vi "CAN_LIN_AsynCall.vi"() -> ()   [LabVIEW 2014]
uses:
  <vilib>/Utility/miscctls.llb/LVPointTypeDef.ctl
  CAN_LIN_FlexRay/TypDef/CAN_LIN_FlexRay_Data.ctl
  TypDef/CAN_LIN_Data.ctl
panel:
  in  "DLL_PATH":path=path "D:/Program Files (x86)/TOSUN/TSMaster/bin/TSMaster.dll"
  out "out put":T1={"Communication message"={"Sender"="", "receiver"="", "message"="", "data"=variant}, "Receive data"="", "error in"={"status"=FALSE, "code"=0, "source"=""}, "Data"={"DLL_PATH"=path "", "Call Array"=["CAN_Demo0", "LIN_Demo0"], "Project_PATH"=path ""}, "AsynCall?"=FALSE}
  in  "选项卡控件":enum32{"CAN", "LIN"}(tab)
  in  "Config":bool
  in  "Connect":bool
  in  "Disconnect":bool
  out "Connect ?":bool
  in  "Creat error":bool
  in  "log":i32(listbox)
  in  "Quit":bool
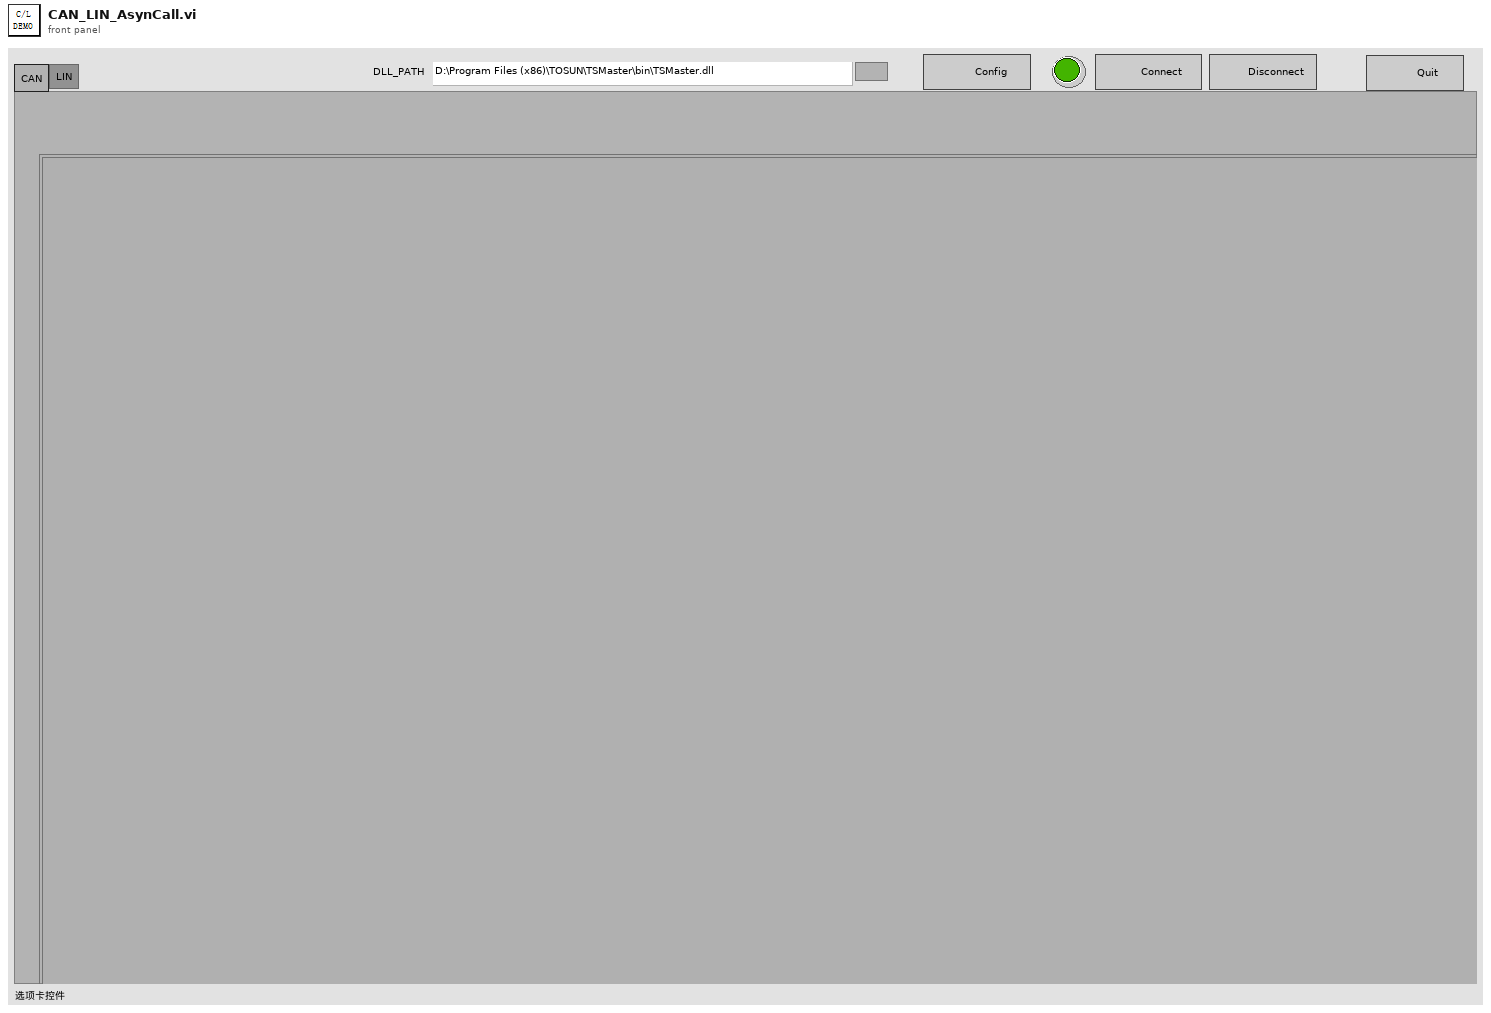
[diagram p1: front panel]
types:
  T1 = typedef "CAN_LIN_Data.ctl" = cluster{"Communication message":cluster{"Sender":string, "receiver":string, "message":string, "data":variant}, "Receive data":string, "error in":errorcluster, "Data":cluster{"DLL_PATH":path, "Call Array":string[], "Project_PATH":path}, "AsynCall?":bool}
  T2 = cluster{"Sender":string, "receiver":string, "message":string, "data":variant}
  T3 = typedef "CAN_LIN_FlexRay_Data.ctl" = cluster{"Communication message":cluster{"Sender":string, "receiver":string, "message":string, "data":variant}, "Receive data":string, "error in":errorcluster, "Data":cluster{"DLL_PATH":path, "Call Array":string[], "Project_PATH":path}, "AsynCall?":bool}
  T4 = typedef "LVPointTypeDef.ctl" = cluster{"Horizontal":i16, "Vertical":i16}
  T5 = enum32{"invalid app kind", "Development System", "Run Time System", "Student Edition", "Embedded LabVIEW", "Evaluation", "Custom"}
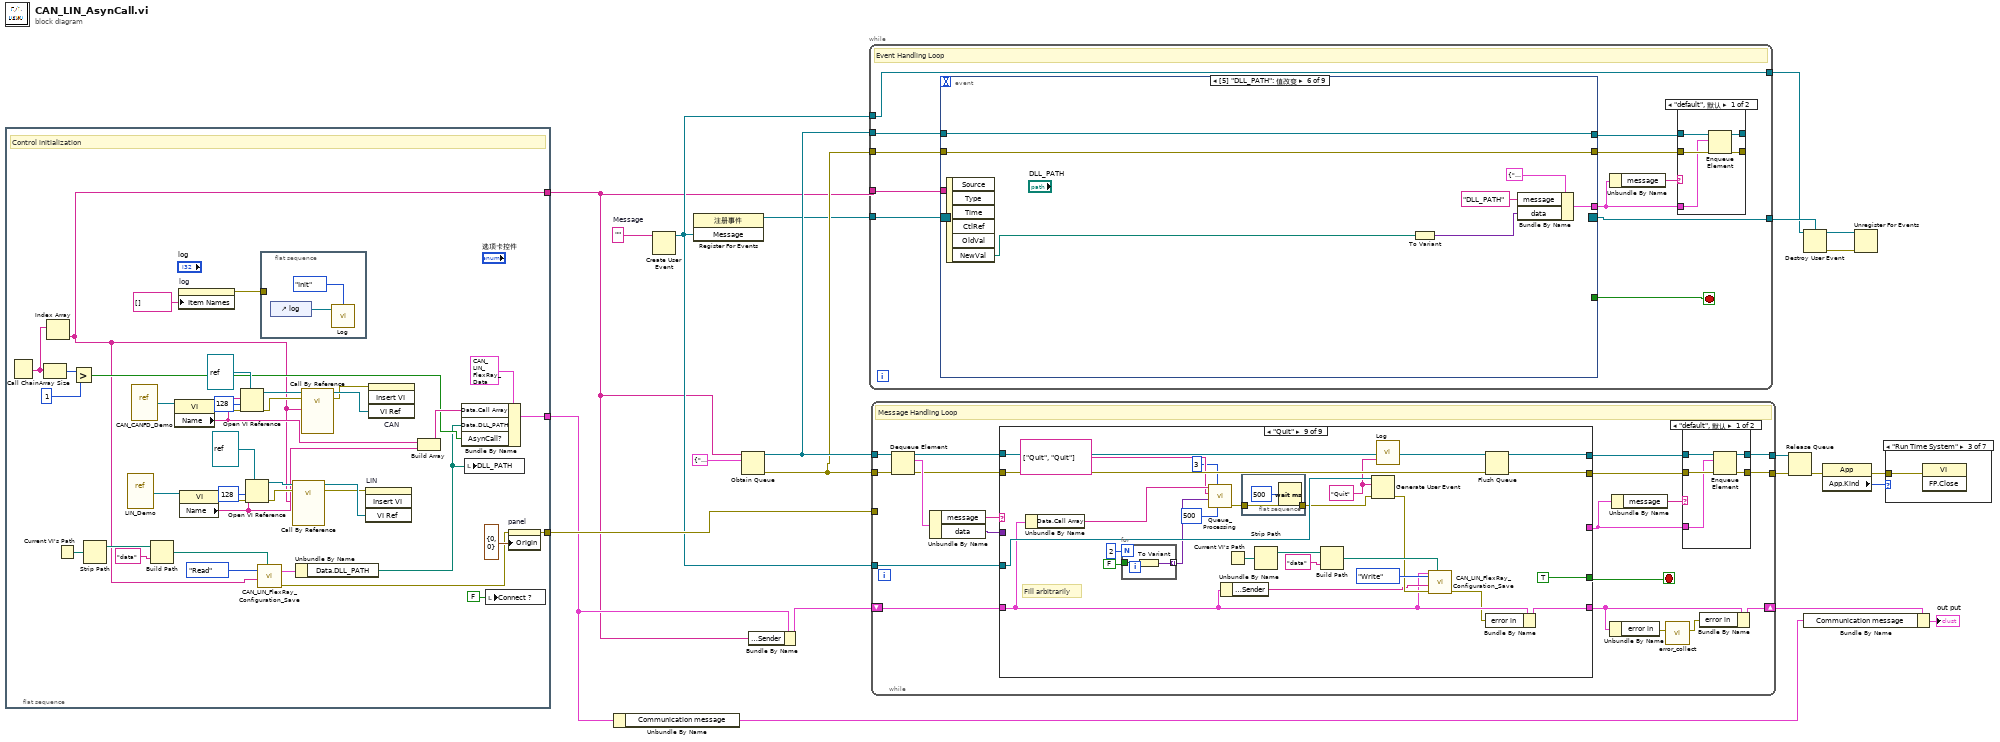
[diagram p0: block diagram]
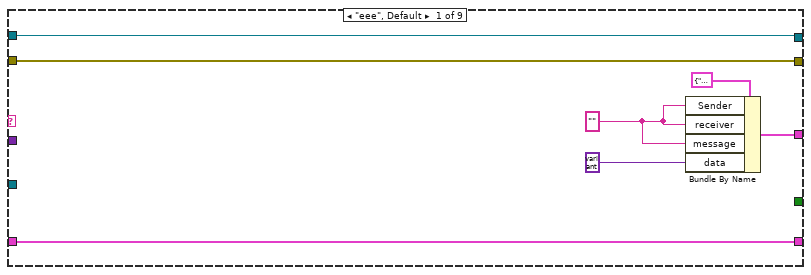
[diagram p9: hidden frame]
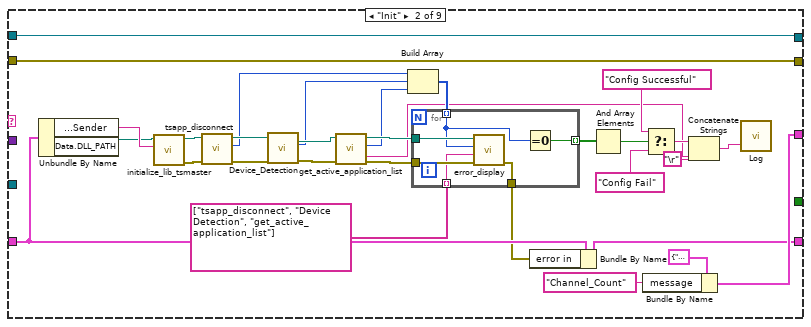
[diagram p10: hidden frame]
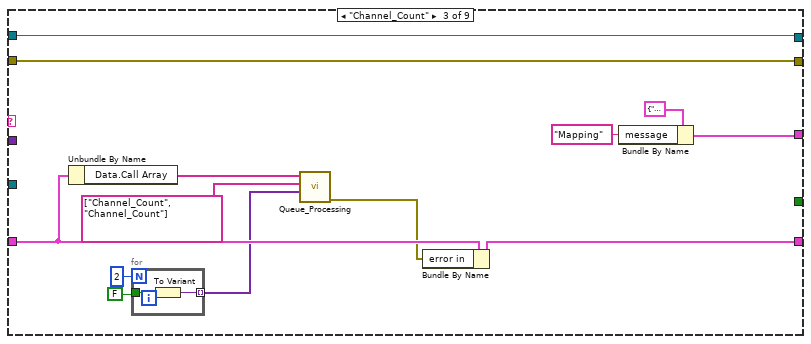
[diagram p11: hidden frame]
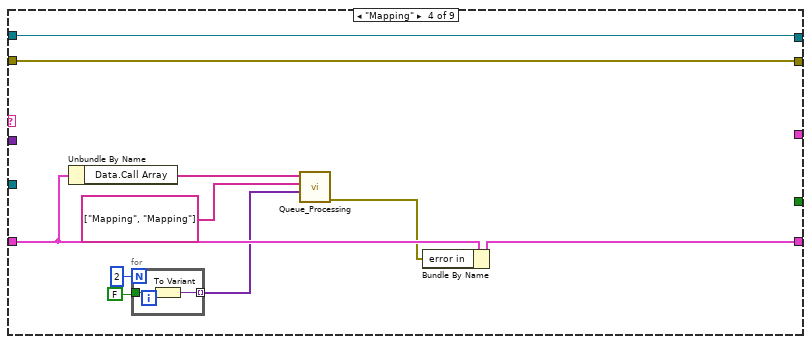
[diagram p12: hidden frame]
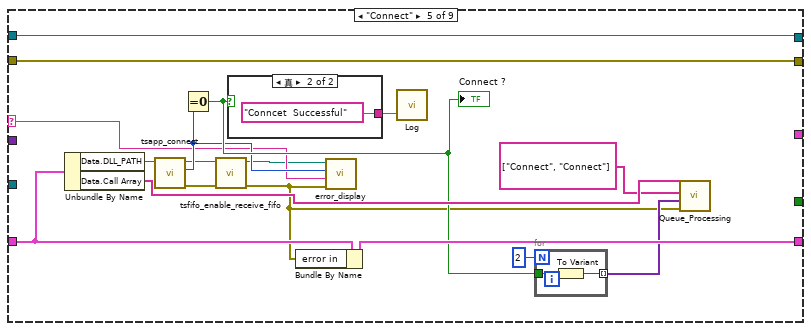
[diagram p13: hidden frame]
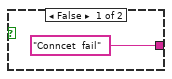
[diagram p14: hidden frame]
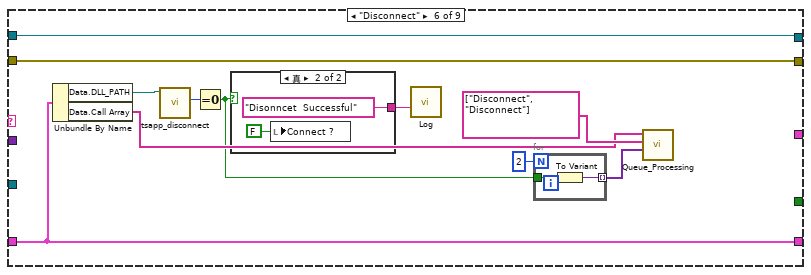
[diagram p15: hidden frame]
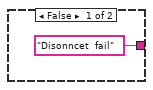
[diagram p16: hidden frame]
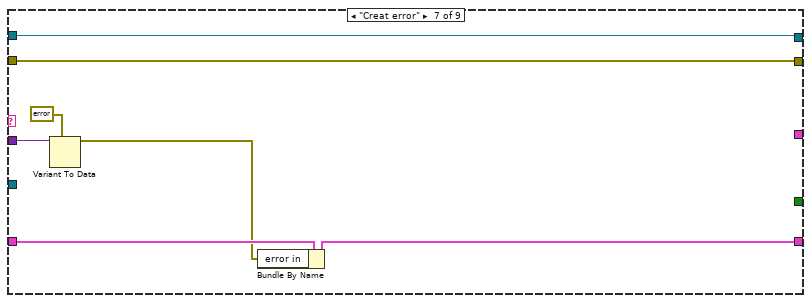
[diagram p17: hidden frame]
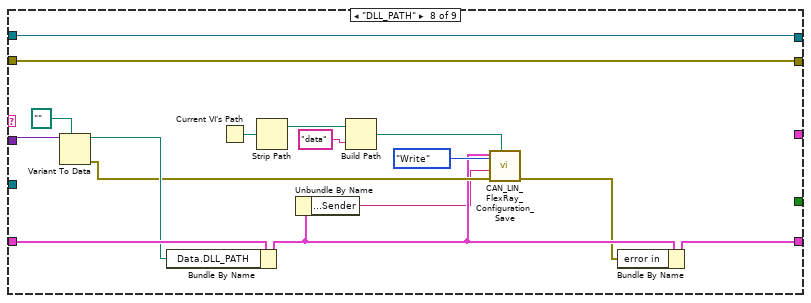
[diagram p18: hidden frame]
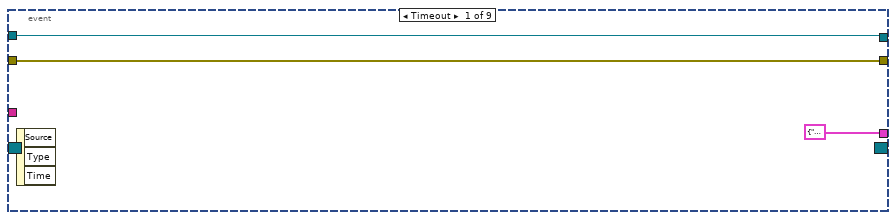
[diagram p20: hidden frame]
diagram:
  w12 = ""  # Message
  n1 = flat-sequence {
    tunnel: [w59] -> w10
    tunnel: [w40] -> w3
    tunnel: [w25] -> w1
    frame #0 {
      # "Control initialization"
      n2 = Call Chain() -> (call chain=w34:string[])
      n3 = Array Size(array=w34) -> (size(s)=w36:i32)
      n4 = Index Array(array=w34) -> (element=w25:string)  [unwired: 1 in]
      n5 = Current VI's Path() -> (path=w30:path)
      n6 = Greater?(x=w36, y=1) -> (0:w33:bool)
      n7 = Strip Path(path=w30) -> (stripped path=w28:path)  [unwired: 1 out]
      n8 = vi-ref "LIN_Demo.vi"() -> (w56:refnum<vi>)
      n9 = vi-ref "CAN_CANFD_Demo.vi"() -> (w45:refnum<vi>)
      n10 = Build Path(base path=w28, name or relative path="data") -> (appended path=w27:path)
      n11 = property class="VI"(reference=w45) -> (error out=w44:errorcluster, "Name"=w38:string)  [unwired: 1 in, 1 out]
      n12 = property on="log" class="LstBox (严格)"("Item Names"=string[] [] ("项名")) -> (error out=w57:errorcluster)  [unwired: 2 in, 1 out]
      n13 = property class="VI"(reference=w56) -> (error out=w43:errorcluster, "Name"=w37:string)  [unwired: 1 in, 1 out]
      n14 = Open VI Reference(type specifier VI Refnum (for type only)=refnum<vi> refnum ("类型说明符VI引用句柄（仅用于类型）"), vi path=w38, options=128 ("选项"), error in (no error)=w44) -> (vi reference=w49:refnum<vi>, error out=w50:errorcluster)  [unwired: 2 in]
      n15 = Open VI Reference(type specifier VI Refnum (for type only)=refnum<vi> refnum ("类型说明符VI引用句柄（仅用于类型）"), vi path=w37, options=128 ("选项"), error in (no error)=w43) -> (vi reference=w54:refnum<vi>, error out=w51:errorcluster)  [unwired: 2 in]
      n16 = call "CAN_LIN_FlexRay_Configuration_Save.vi"("path"=w27, "Config Name"=w25, "Read/Write"=enum16{"Read", "Write"}."Read") -> ("error in (no error)"=w23:errorcluster, "Data out"=w24:T3)  [unwired: 6 in, 1 out]
      n17 = flat-sequence {
        tunnel: w57 -> [_]
        frame #0 {
          n18 = control-ref of="log"() -> (w61:refnum<vi>)
          n19 = call "Log.vi"("Method"=enum16{"Init", "Log"}."Init", "ListBox in"=w61) -> ()  [unwired: 2 in]
        }
      }
      n20 = call-by-ref "?"(reference=w54, error in=w51, "Sender"=w25) -> (reference out=w53:refnum<vi>, error out=w52:errorcluster)  [unwired: 11 in]
      n21 = Unbundle By Name(w24) -> ("Data.DLL_PATH"=w22:path)
      n22 = call-by-ref "?"(reference=w49, error in=w50, "Sender"=w25) -> (reference out=w47:refnum<vi>, error out=w46:errorcluster)  [unwired: 11 in]
      n23 = invoke on="LIN" class="SubPnl" method="Insert VI"(error in=w52, "VI Ref"=w53) -> ()  [unwired: 2 in, 4 out]
      n24 = invoke on="CAN" class="SubPnl" method="Insert VI"(error in=w46, "VI Ref"=w47) -> ()  [unwired: 2 in, 4 out]
      n25 = Build Array(w38, w37) -> (w39:string[])
      n26 = Bundle By Name(cluster=T3 {"Communication message"={"Sender"="", "receiver"="", "message"="", "data"=variant}, "Receive data"="", "error in"={"status"=FALSE, "code"=0, "source"=""}, "Data"={"DLL_PATH"=path "", "Call Array"=["CAN_Demo0", "LIN_Demo0"], "Project_PATH"=path ""}, "AsynCall?"=FALSE} ("Data"), "Data.Call Array"=w39, "Data.DLL_PATH"=w22, "AsynCall?"=w33) -> (w40:T3)
      n27 = local write "DLL_PATH"(w22) -> ()
      n28 = local write "Connect ?"(FALSE ("Connect ?")) -> ()
      n29 = property on="panel" class="Pane"(error in=w23, "Origin"=T4 {"Horizontal"=0, "Vertical"=0} ("原点")) -> (error out=w59:errorcluster)  [unwired: 1 in, 1 out]
    }
  }
  n30 = Unbundle By Name(w3) -> ("Communication message"=w4:T2)
  n31 = Create User Event(user event datatype=w12) -> (user event=w7:refnum<user-event>)  [unwired: 1 in, 1 out]
  n32 = register-events(w7) -> (reference out=w11:refnum<event-registration>)  [unwired: 2 in, 1 out]
  n33 = Obtain Queue(name (unnamed)=w1, element data type=T2 {"Sender"="", "receiver"="", "message"="", "data"=variant} ("Communication message")) -> (queue out=w21:refnum<queue>, error out=w14:errorcluster)  [unwired: 3 in, 1 out]
  n34 = Bundle By Name(cluster=w3, "Communication message.Sender"=w1) -> (w13:T3)
  n35 = while {
    tunnel: w21 -> [w72]
    tunnel: w14 -> [w70]
    tunnel: w1 -> [w66]
    tunnel: w11 -> [w65]
    tunnel: [w64] -> w9
    tunnel: w7 -> [w63]
    tunnel: [w63] -> w6
    stop <- w73 stop-if-true
    # "Event Handling Loop"
    n36 = event shown="[5] \"DLL_PATH\": 值改变" {
      selector: w65 -> [_ _ _ _ _ _ _ _ _]
      dyn-events: [_ _ _ _ _ _ _ _ _] -> w64
      timeout: _ -> [_ _ _ _ _ _ _ _ _]
      tunnel: [_ _ w90 w95 _ _ _ _ _] -> w73
      tunnel: w72 -> [w83 w88 w93 w98 w105 w112 w117 w122 w127]
      tunnel: [w83 w88 w93 w96 w105 w112 w117 w122 w127] -> w71
      tunnel: [T2 {"Sender"="", "receiver"="", "message"="", "data"=variant} ("Communication message") w86 _ _ w101 w108 w113 w118 w123] -> w68
      tunnel: [w82 w84 w89 w94 w104 w111 w116 w121 w126] -> w69
      tunnel: w70 -> [w82 w84 w89 w94 w104 w111 w116 w121 w126]
      tunnel: w66 -> [_ _ _ _ _ _ _ _ _]
      event Timeout {
        n37 = event-data() -> ()  [unwired: 1 in, 3 out]
      }
      event "Quit": Value Change {
        n38 = event-data() -> ()  [unwired: 1 in, 6 out]
        n39 = Bundle By Name(cluster=T2 {"Sender"="", "receiver"="", "message"="", "data"=variant} ("Communication message"), "message"="Quit" ("Sender")) -> (w86:T2)
      }
      event User Event {
        n40 = event-data() -> ("Message"=w92:string)  [unwired: 1 in]
        n41 = Equal?(x=w92, y="Quit") -> (x = y?=w90:bool)
      }
      event Panel Close? {
        w95 = TRUE ("放弃？")
        n42 = event-data() -> ()  [unwired: 1 in, 4 out]
        n43 = Enqueue Element(queue=w98, element=T2 {"Sender"="", "receiver"="", "message"="Quit", "data"=variant} ("Communication message")) -> (queue out=w96:refnum<queue>)  [unwired: 2 in, 2 out]
        n44 = event-data("Discard?"=w95) -> ()  [unwired: 1 in, 1 out]
      }
      event "Creat error": Value Change {
        n45 = event-data() -> ()  [unwired: 1 in, 6 out]
        n46 = To Variant(anything=errorcluster {"status"=TRUE, "code"=709394, "source"="This is a error demo"}) -> (Variant=w99:variant)
        n47 = Bundle By Name(cluster=T2 {"Sender"="", "receiver"="", "message"="", "data"=variant} ("Communication message"), "message"="Creat error" ("Sender"), "data"=w99) -> (w101:T2)
      }
      event "DLL_PATH": Value Change {
        n48 = event-data() -> ("NewVal"=w106:path)  [unwired: 1 in, 5 out]
        n49 = To Variant(anything=w106) -> (Variant=w107:variant)
        n50 = Bundle By Name(cluster=T2 {"Sender"="", "receiver"="", "message"="", "data"=variant} ("Communication message"), "message"="DLL_PATH" ("Sender"), "data"=w107) -> (w108:T2)
      }
      event "Config": Value Change {
        n51 = event-data() -> ()  [unwired: 1 in, 6 out]
        n52 = Bundle By Name(cluster=T2 {"Sender"="", "receiver"="", "message"="", "data"=variant} ("Communication message"), "message"="Init" ("Sender")) -> (w113:T2)
      }
      event "Connect": Value Change {
        n53 = event-data() -> ()  [unwired: 1 in, 6 out]
        n54 = Bundle By Name(cluster=T2 {"Sender"="", "receiver"="", "message"="", "data"=variant} ("Communication message"), "message"="Connect" ("Sender")) -> (w118:T2)
      }
      event "Disconnect": Value Change {
        n55 = event-data() -> ()  [unwired: 1 in, 6 out]
        n56 = Bundle By Name(cluster=T2 {"Sender"="", "receiver"="", "message"="", "data"=variant} ("Communication message"), "message"="Disconnect" ("Sender")) -> (w123:T2)
      }
    }
    n57 = Unbundle By Name(w68) -> ("message"=w67:string)
    n58 = case shown="\"default\", 默认" w67 {
      tunnel: w71 -> [w78 w80]
      tunnel: w69 -> [w77 w79]
      tunnel: w68 -> [w76 _]
      tunnel: [w75 w80] -> _
      tunnel: [w74 w79] -> _
      frame "default", Default {
        n59 = Enqueue Element(queue=w78, element=w76, error in (no error)=w77) -> (queue out=w75:refnum<queue>, error out=w74:errorcluster)  [unwired: 1 in, 1 out]
      }
      frame "" {
      }
    }
  }
  n60 = while {
    tunnel: w21 -> [w147]
    tunnel: w14 -> [w146]
    tunnel: [w138] -> w20
    tunnel: [w137] -> w19
    shift-right: [w129] -> w5
    shift-left: w13 -> [w133]
    tunnel: w10 -> [_]
    tunnel: w7 -> [w132]
    stop <- w136 stop-if-true
    # "Message Handling Loop"
    n61 = Dequeue Element(queue=w147, error in (no error)=w146) -> (queue out=w143:refnum<queue>, element=w145:T2, error out=w142:errorcluster)  [unwired: 1 in, 1 out]
    n62 = Unbundle By Name(w145) -> ("message"=w144:string, "data"=w139:variant)
    n63 = case shown="\"Quit\"" w144 {
      selector: w144 -> [_ _ _ _ w229 _ _ _ _]
      tunnel: [w161 w192 w211 w223 w242 w257 w269 w285 w310] -> w141
      tunnel: w143 -> [w161 w192 w211 w223 w242 w257 w269 w285 w309]
      tunnel: w142 -> [w160 w191 w210 w222 w241 w256 w268 w284 w307]
      tunnel: [w160 w191 w210 w222 w241 w256 w268 w284 w308] -> w140
      tunnel: w139 -> [_ _ _ _ _ _ w266 w282 _]
      tunnel: [_ _ _ _ _ _ _ _ TRUE] -> w136
      tunnel: [w158 w167 w199 _ _ _ _ _ _] -> w135
      tunnel: [w155 w166 w207 w219 w237 w253 w264 w271 w288] -> w131
      tunnel: w133 -> [w155 w170 w209 w221 w239 w253 w267 w283 w289]
      tunnel: w132 -> [_ _ _ _ _ _ _ _ w306]
      frame "eee", Default {
        w156 = ""
        n64 = Bundle By Name(cluster=T2 {"Sender"="", "receiver"="", "message"="", "data"=variant} ("Communication message"), "Sender"=w156, "receiver"=w156, "message"=w156, "data"=variant) -> (w158:T2)
      }
      frame "Init" {
        n65 = Unbundle By Name(w170) -> ("Communication message.Sender"=w190:string, "Data.DLL_PATH"=w189:path)
        n66 = call "initialize_lib_tsmaster.vi"("AppName"=w190, "Path input"=w189) -> ("error output"=w187:errorcluster, "Path output"=w188:path)  [unwired: 8 in]
        n67 = call "tsapp_disconnect.vi"("error in (no error)"=w187, "Path"=w188) -> ("error output"=w185:errorcluster, "retuen"=w180:i32, "Path output"=w186:path)  [unwired: 7 in]
        n68 = call "Device_Detection.vi"("error in (no error)"=w185, "Path"=w186) -> ("error out"=w183:errorcluster, "retuen"=w179:i32, "Path output"=w184:path)  [unwired: 7 in]
        n69 = call "get_active_application_list.vi"("error in"=w183, "path in"=w184) -> ("error out"=w181:errorcluster, "ATSMasterAppNames"=w162:string, "return"=w178:i32, "path out"=w182:path)  [unwired: 6 in]
        n70 = Build Array(w180, w179, w178) -> (w177:i32[])
        n71 = for {
          tunnel: w182 -> [w198]
          tunnel: w181 -> [w197]
          tunnel: w177 -> [w195] mode=indexing
          tunnel: string[] ["tsapp_disconnect", "Device Detection", "get_active_application_list"] -> [w196] mode=indexing
          tunnel: [w194] -> w175 mode=indexing
          tunnel: [w193] -> w165
          n72 = call "error_display.vi"("error in"=w197, "Action name"=w196, "return"=w195, "DLL path"=w198) -> ("error out"=w193:errorcluster)  [unwired: 6 in, 1 out]
          n73 = Equal To 0?(x=w195) -> (x = 0?=w194:bool)
        }
        n74 = Bundle By Name(cluster=w170, "error in"=w165) -> (w166:T3)
        n75 = And Array Elements(Boolean array=w175) -> (logical AND=w174:bool)
        n76 = Bundle By Name(cluster=T2 {"Sender"="", "receiver"="", "message"="", "data"=variant} ("Communication message"), "message"="Channel_Count") -> (w167:T2)
        n77 = Select(t="Config Successful", s=w174, f="Config Fail") -> (s? t:f=w171:string)
        n78 = Concatenate Strings(w171, "\r", w162) -> (w164:string)
        n79 = call "Log.vi"("Data"=w164) -> ()  [unwired: 3 in]
      }
      frame "Channel_Count" {
        n80 = Unbundle By Name(w209) -> ("Data.Call Array"=w208:string[])
        n81 = for {
          N: 2 -> [_]
          tunnel: [w213] -> w202 mode=indexing
          tunnel: FALSE -> [w212]
          n82 = To Variant(anything=w212) -> (Variant=w213:variant)
        }
        n83 = call "Queue_Processing.vi"("Data Array"=w202, "Cmd Array"=string[] ["Channel_Count", "Channel_Count"], "Call Array"=w208) -> ("error out"=w206:errorcluster)  [unwired: 8 in]
        n84 = Bundle By Name(cluster=w209, "error in"=w206) -> (w207:T3)
        n85 = Bundle By Name(cluster=T2 {"Sender"="", "receiver"="", "message"="", "data"=variant} ("Communication message"), "message"="Mapping") -> (w199:T2)
      }
      frame "Mapping" {
        n86 = Unbundle By Name(w221) -> ("Data.Call Array"=w220:string[])
        n87 = for {
          N: 2 -> [_]
          tunnel: [w225] -> w214 mode=indexing
          tunnel: FALSE -> [w224]
          n88 = To Variant(anything=w224) -> (Variant=w225:variant)
        }
        n89 = call "Queue_Processing.vi"("Data Array"=w214, "Cmd Array"=string[] ["Mapping", "Mapping"], "Call Array"=w220) -> ("error out"=w218:errorcluster)  [unwired: 8 in]
        n90 = Bundle By Name(cluster=w221, "error in"=w218) -> (w219:T3)
      }
      frame "Connect" {
        n91 = Unbundle By Name(w239) -> ("Data.DLL_PATH"=w238:path, "Data.Call Array"=w236:string[])
        n92 = call "tsapp_connect.vi"("Path"=w238) -> ("error out"=w227:errorcluster, "retuen"=w231:i32, "Path output"=w228:path)  [unwired: 8 in]
        n93 = Equal To 0?(x=w231) -> (x = 0?=w232:bool)
        "Connect ?" <- w232
        n94 = call "tsfifo_enable_receive_fifo.vi"("error in (no error)"=w227, "Path"=w228) -> ("error out"=w230:errorcluster, "Path output"=w226:path)  [unwired: 8 in]
        n95 = case shown="真" w232 {
          tunnel: ["Conncet  fail" ("消息") "Conncet  Successful" ("消息")] -> w240
          frame False {
          }
          frame True {
          }
        }
        n96 = Bundle By Name(cluster=w239, "error in"=w230) -> (w237:T3)
        n97 = call "error_display.vi"("error in"=w230, "Action name"=w229, "return"=w231, "DLL path"=w226) -> ()  [unwired: 6 in, 2 out]
        n98 = call "Log.vi"("Data"=w240) -> ()  [unwired: 3 in]
        n99 = for {
          N: 2 -> [_]
          tunnel: w232 -> [w244]
          tunnel: [w243] -> w234 mode=indexing
          n100 = To Variant(anything=w244) -> (Variant=w243:variant)
        }
        n101 = call "Queue_Processing.vi"("error in (no error)"=w230, "Data Array"=w234, "Cmd Array"=string[] ["Connect", "Connect"], "Call Array"=w236) -> ()  [unwired: 7 in, 1 out]
      }
      frame "Disconnect" {
        n102 = Unbundle By Name(w253) -> ("Data.DLL_PATH"=w255:path, "Data.Call Array"=w248:string[])
        n103 = call "tsapp_disconnect.vi"("Path"=w255) -> ("retuen"=w252:i32)  [unwired: 8 in, 2 out]
        n104 = Equal To 0?(x=w252) -> (x = 0?=w247:bool)
        n105 = case shown="真" w247 {
          tunnel: ["Disonncet  fail" ("消息") "Disonncet  Successful" ("消息")] -> w254
          frame False {
          }
          frame True {
            n106 = local write "Connect ?"(FALSE ("Connect ?")) -> ()
          }
        }
        n107 = call "Log.vi"("Data"=w254) -> ()  [unwired: 3 in]
        n108 = for {
          N: 2 -> [_]
          tunnel: [w259] -> w250 mode=indexing
          tunnel: w247 -> [w258]
          n109 = To Variant(anything=w258) -> (Variant=w259:variant)
        }
        n110 = call "Queue_Processing.vi"("Data Array"=w250, "Cmd Array"=string[] ["Disconnect", "Disconnect"], "Call Array"=w248) -> ()  [unwired: 8 in, 1 out]
      }
      frame "Creat error" {
        n111 = Variant To Data(type=errorcluster {"status"=FALSE, "code"=0, "source"=""} ("error out"), Variant=w266) -> (data=w263:errorcluster)  [unwired: 1 in, 1 out]
        n112 = Bundle By Name(cluster=w267, "error in"=w263) -> (w264:T3)
      }
      frame "DLL_PATH" {
        n113 = Variant To Data(type=path "" ("新值"), Variant=w282) -> (data=w280:path, error out=w274:errorcluster)  [unwired: 1 in]
        n114 = Bundle By Name(cluster=w283, "Data.DLL_PATH"=w280) -> (w273:T3)
        n115 = Current VI's Path() -> (path=w279:path)
        n116 = Strip Path(path=w279) -> (stripped path=w277:path)  [unwired: 1 out]
        n117 = Unbundle By Name(w273) -> ("Communication message.Sender"=w272:string)
        n118 = Build Path(base path=w277, name or relative path="data") -> (appended path=w276:path)
        n119 = call "CAN_LIN_FlexRay_Configuration_Save.vi"("path"=w276, "error in (no error)"=w274, "Config Name"=w272, "Read/Write"=enum16{"Read", "Write"}."Write", "Data"=w273) -> ("error in (no error)"=w270:errorcluster)  [unwired: 4 in, 2 out]
        n120 = Bundle By Name(cluster=w273, "error in"=w270) -> (w271:T3)
      }
      frame "Quit" {
        w305 = "Quit" ("y")
        # "Fill arbitrarily"
        n121 = Unbundle By Name(w289) -> ("Data.Call Array"=w302:string[])
        n122 = for {
          N: 2 -> [_]
          tunnel: [w313] -> w299 mode=indexing
          tunnel: FALSE -> [w312]
          n123 = To Variant(anything=w312) -> (Variant=w313:variant)
        }
        n124 = call "Queue_Processing.vi"("Delay(ms)"=u32 500, "loop val"=3, "Data Array"=w299, "Cmd Array"=string[] ["Quit", "Quit"], "Call Array"=w302) -> ("error out"=w304:errorcluster)  [unwired: 6 in]
        n125 = Unbundle By Name(w289) -> ("Communication message.Sender"=w290:string)
        n126 = Current VI's Path() -> (path=w296:path)
        n127 = flat-sequence {
          tunnel: w304 -> [w314]
          tunnel: [w314] -> w303
          frame #0 {
            n128 = Wait (ms)(milliseconds to wait=u32 500 ("等待时间（毫秒）")) -> ()  [unwired: 1 out]
          }
        }
        n129 = Strip Path(path=w296) -> (stripped path=w294:path)  [unwired: 1 out]
        n130 = Build Path(base path=w294, name or relative path="data") -> (appended path=w293:path)
        n131 = Generate User Event(user event=w306, event data cluster=w305, error in=w303) -> (error out=w291:errorcluster)  [unwired: 1 in, 1 out]
        n132 = call "Log.vi"("Data"=w305) -> ()  [unwired: 3 in]
        n133 = call "CAN_LIN_FlexRay_Configuration_Save.vi"("path"=w293, "error in (no error)"=w291, "Config Name"=w290, "Read/Write"=enum16{"Read", "Write"}."Write", "Data"=w289) -> ("error in (no error)"=w287:errorcluster)  [unwired: 4 in, 2 out]
        n134 = Bundle By Name(cluster=w289, "error in"=w287) -> (w288:T3)
        n135 = Flush Queue(queue=w309, error in (no error)=w307) -> (queue out=w310:refnum<queue>, error out=w308:errorcluster)  [unwired: 1 out]
      }
    }
    n136 = Unbundle By Name(w131) -> ("error in"=w130:errorcluster)
    n137 = Unbundle By Name(w135) -> ("message"=w134:string)
    n138 = call "error_collect.vi"("error in (no error)"=w130) -> ("error IO"=w128:errorcluster)  [unwired: 10 in]
    n139 = case shown="\"default\", 默认" w134 {
      tunnel: w141 -> [w152 w154]
      tunnel: w140 -> [w151 w153]
      tunnel: w135 -> [w150 _]
      tunnel: [w149 w154] -> w138
      tunnel: [w148 w153] -> w137
      frame "default", Default {
        n140 = Enqueue Element(queue=w152, element=w150, error in (no error)=w151) -> (queue out=w149:refnum<queue>, error out=w148:errorcluster)  [unwired: 1 in, 1 out]
      }
      frame "" {
      }
    }
    n141 = Bundle By Name(cluster=w131, "error in"=w128) -> (w129:T3)
  }
  n142 = Release Queue(queue=w20, error in (no error)=w19) -> (error out=w18:errorcluster)  [unwired: 1 in, 2 out]
  n143 = Destroy User Event(user event=w6) -> (error out=w8:errorcluster)  [unwired: 1 in]
  n144 = Bundle By Name(cluster=w5, "Communication message"=w4) -> (→"out put":T3)
  n145 = property class="App"(error in=w18) -> (error out=w17:errorcluster, "App.Kind"=w16:T5)  [unwired: 1 in, 1 out]
  n146 = Unregister For Events(event registration refnum=w9, error in=w8) -> ()  [unwired: 1 out]
  n147 = case shown="\"Run Time System\"" w16 {
    tunnel: w17 -> [_ _ w316 _ _ _ _]
    frame "invalid app kind", Default {
    }
    frame "Development System" {
    }
    frame "Run Time System" {
      n148 = invoke class="VI" method="FP.Close"(error in=w316) -> ()  [unwired: 2 in, 3 out]
    }
    frame "Student Edition" {
    }
    frame "Embedded LabVIEW" {
    }
    frame "Evaluation" {
    }
    frame "Custom" {
    }
  }
